vi "Settings Dialog.vi"(8 "error in (no error)":errorcluster, 11 "Settings in":T1={"Hardware Configuration"={"DAQmx Channel"="", "Max Input"=10.0, "Min Input"=-10.0, "Sample Rate"=1000.0, "DAQmx Task"=""}, "Logging Configuration"={"Log File Base Path"=path "", "TDMS File Reference"=refnum, "Samples to Save"=0, "Trigger - Time"=0, "Trigger - Threshold"=0.0, "Trigger - Channel"=0, "Enable Time Trigger"=FALSE, "Enable Threshold Trigger"=FALSE, "Always Log"=FALSE}}) -> (0 "error out":errorcluster, 1 "Cancelled?":bool=TRUE, 2 "UI Refresh Needed?":bool, 3 "Settings out":T1={"Hardware Configuration"={"DAQmx Channel"="", "Max Input"=10.0, "Min Input"=-10.0, "Sample Rate"=1000.0, "DAQmx Task"=""}, "Logging Configuration"={"Log File Base Path"=path "C:/Users/jpassiak/Documents/LabVIEW Data/Logged Data.tdms", "TDMS File Reference"=refnum, "Samples to Save"=0, "Trigger - Time"=0, "Trigger - Threshold"=0.0, "Trigger - Channel"=0, "Enable Time Trigger"=FALSE, "Enable Threshold Trigger"=FALSE, "Always Log"=FALSE}})   [LabVIEW 2015, in "Settings.lvlib"]
doc: "Dialog for selecting user specified settings."
uses:
  Settings.lvlib
  Settings.ctl
  Acquisition/Hardware Configuration.ctl
  Logging/Logging Configuration.ctl
  <vilib>/Utility/xml.llb/Write to XML File(string).vi
  Acquisition/Acquisition.lvlib
  Logging/Logging.lvlib
panel:
  in  "Log when triggered":bool
  in  "Trigger Channel":u32
  in  "Samples to Log":u32=500 min=1
  in  "Trigger Threshold (V)":dbl=2.0
  in  "Trigger Time (min)":u32=1
  in  "Enable Threshold Trigger (V):":bool
  in  "Enable Time Trigger (min):":bool
  in  "Always Log":bool
  in  "Sample Rate":dbl=1000.0
  in  "Minimum Input":dbl=-10.0
  in  "Maximum Input":dbl=10.0
  in  "DAQmx Channel":tag="Dev1/ai0"
  in  "Log File Path":path
  in  "Cancel Button":bool
  in  "OK Button":bool
  # "Acquisition"
  # "Non visible portion of dialog (needed for connector pane)."
  # "Trigger"
  # "Logging"
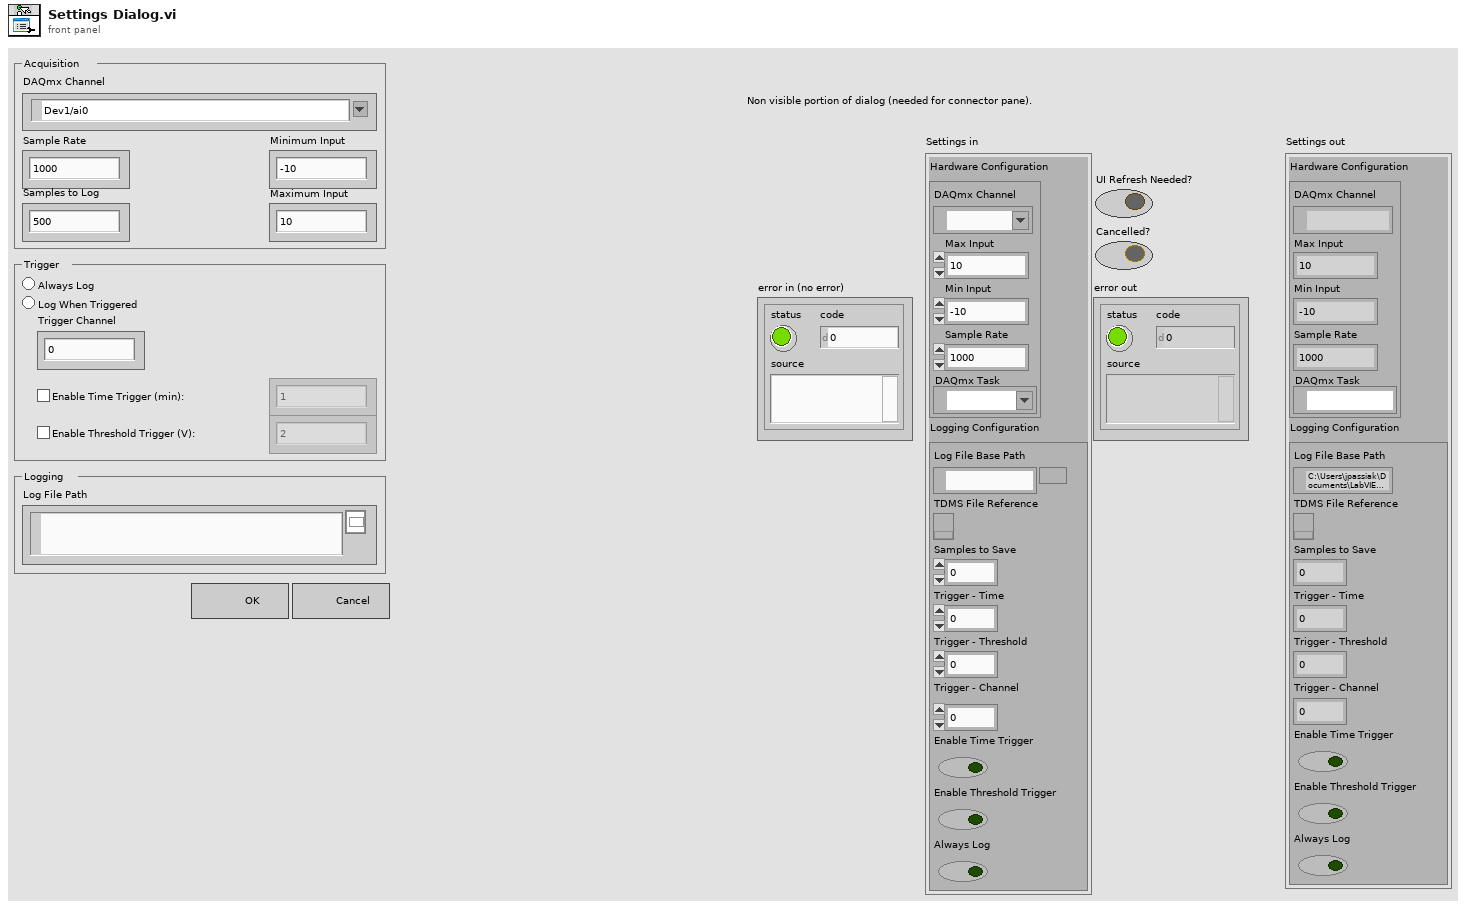
[diagram p1: front panel]
types:
  T1 = typedef "Settings.lvlib/Settings.ctl" = cluster{"Hardware Configuration":T2, "Logging Configuration":T3}
  T2 = typedef "Acquisition.lvlib/Hardware Configuration.ctl" = cluster{"DAQmx Channel":tag, "Max Input":dbl, "Min Input":dbl, "Sample Rate":dbl, "DAQmx Task":refnum<k21>}
  T3 = typedef "Logging.lvlib/Logging Configuration.ctl" = cluster{"Log File Base Path":path, "TDMS File Reference":refnum<k34>, "Samples to Save":u32, "Trigger - Time":u32, "Trigger - Threshold":dbl, "Trigger - Channel":u32, "Enable Time Trigger":bool, "Enable Threshold Trigger":bool, "Always Log":bool}
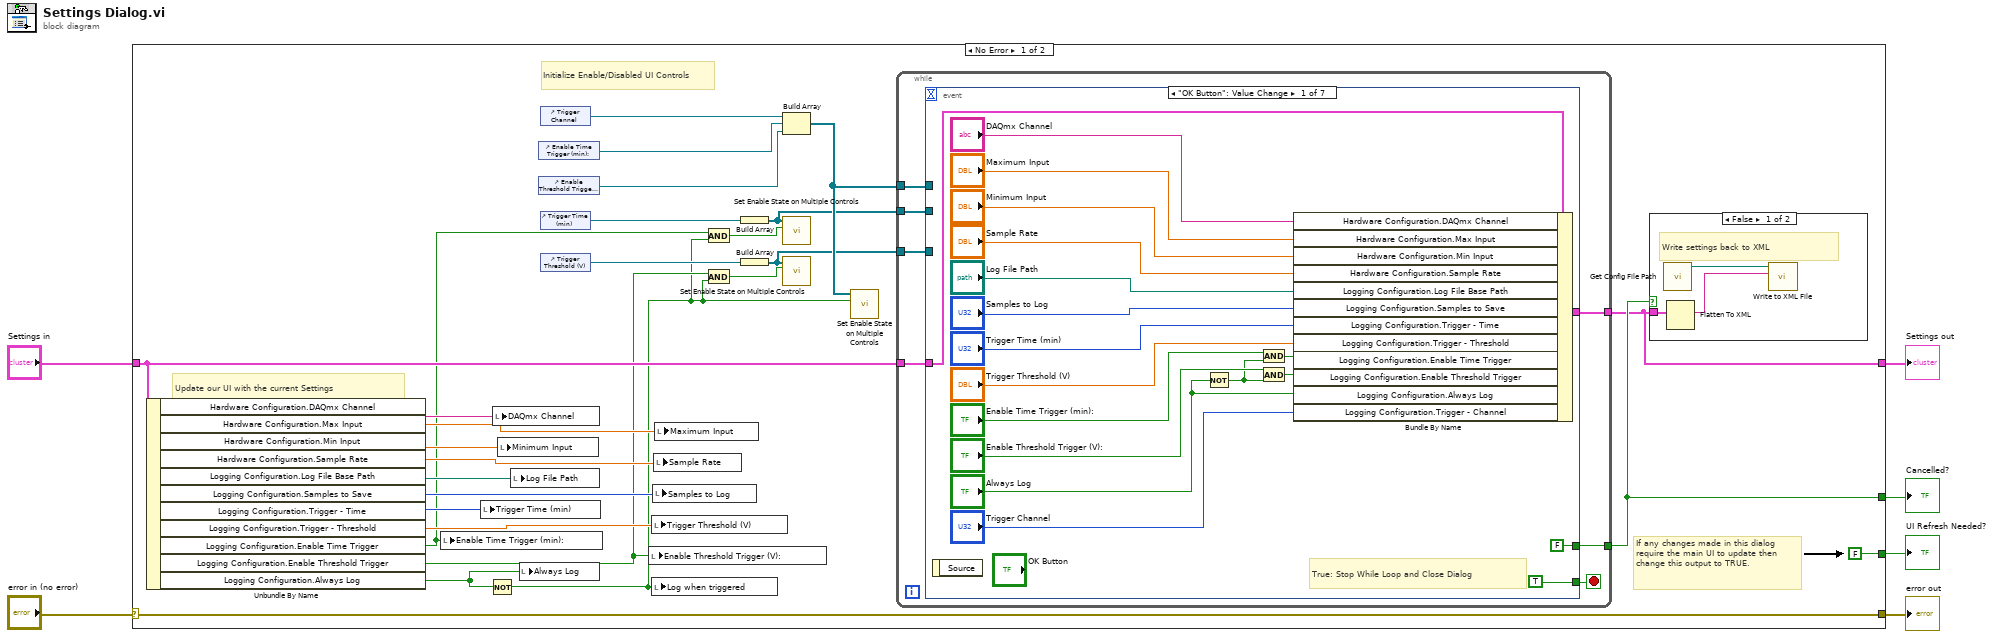
[diagram p0: block diagram]
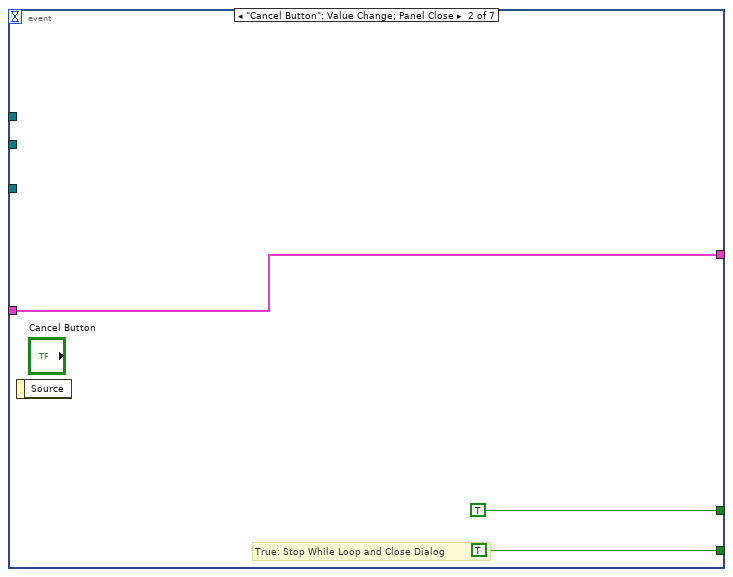
[diagram p2: hidden frame]
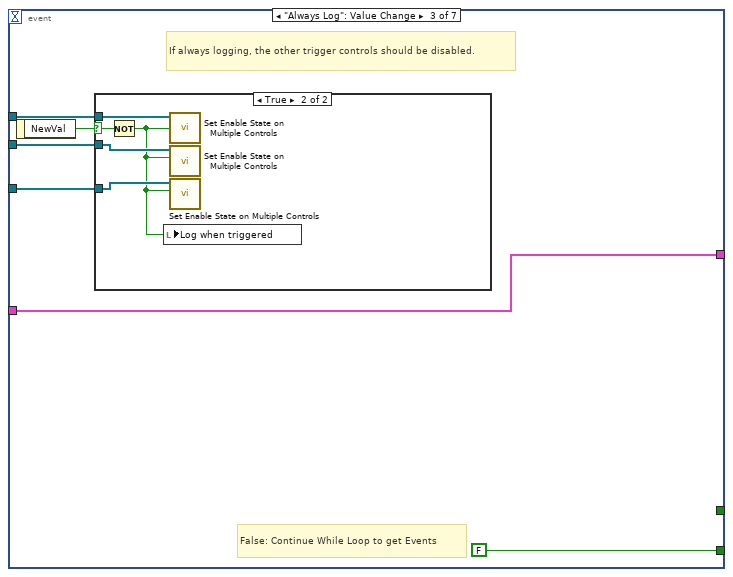
[diagram p3: hidden frame]
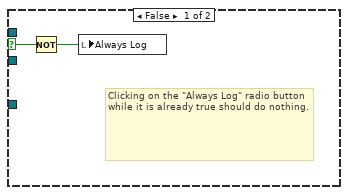
[diagram p4: hidden frame]
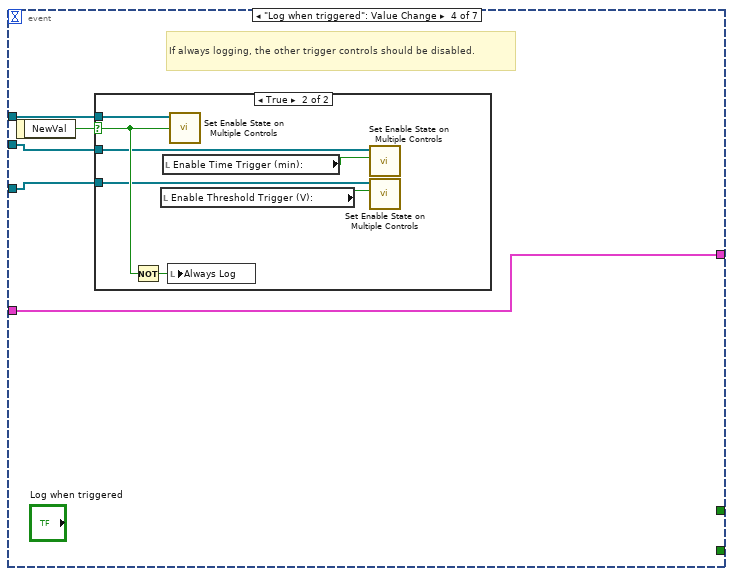
[diagram p5: hidden frame]
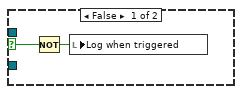
[diagram p6: hidden frame]
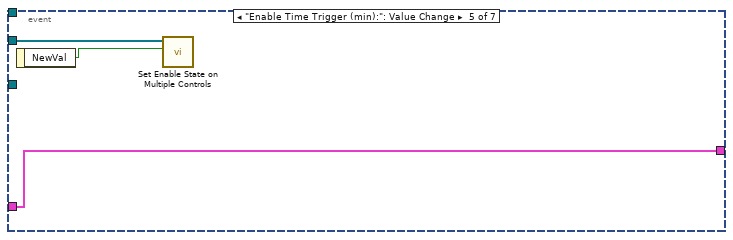
[diagram p7: hidden frame]
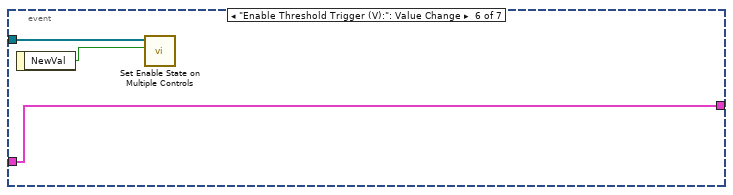
[diagram p8: hidden frame]
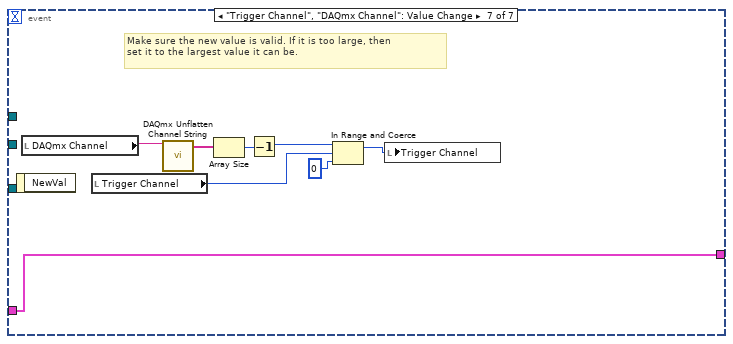
[diagram p9: hidden frame]
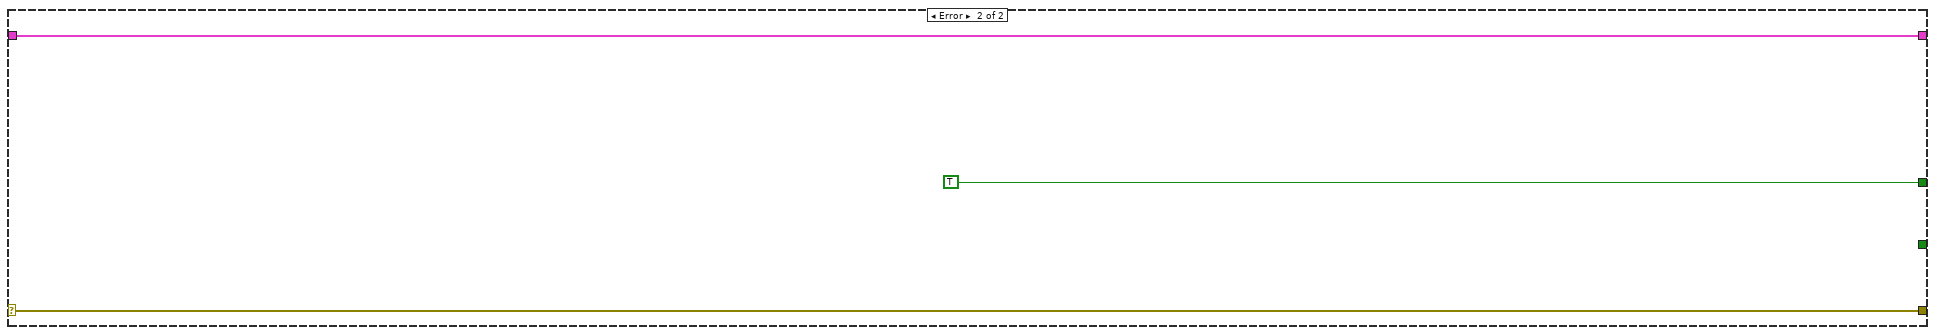
[diagram p11: hidden frame]
diagram:
  n1 = case shown="No Error" "error in (no error)" {
    selector: "error in (no error)" -> [w33 w109]
    tunnel: [w33 w109] -> w6
    tunnel: "Settings in" -> [w19 w108]
    tunnel: [w30 w108] -> w4
    tunnel: [FALSE ("UI Refresh Needed?") _] -> w3
    tunnel: [w31 TRUE ("UI Refresh Needed?")] -> w2
    frame No Error {
      # "Update our UI with the current Settings"
      # "Initialize Enable/Disabled UI Controls"
      # "If any changes made in this dialog require the main UI to update then change this output to TRUE."
      n2 = Unbundle By Name(w19) -> ("Hardware Configuration.DAQmx Channel"=w26:tag, "Hardware Configuration.Max Input"=w27:dbl, "Hardware Configuration.Min Input"=w28:dbl, "Hardware Configuration.Sample Rate"=w29:dbl, "Logging Configuration.Log File Base Path"=w25:path, "Logging Configuration.Samples to Save"=w24:u32, "Logging Configuration.Trigger - Time"=w23:u32, "Logging Configuration.Trigger - Threshold"=w22:dbl, "Logging Configuration.Enable Time Trigger"=w11:bool, "Logging Configuration.Enable Threshold Trigger"=w10:bool, "Logging Configuration.Always Log"=w21:bool)
      n3 = local write "Enable Time Trigger (min):"(w11) -> ()
      n4 = local write "Trigger Time (min)"(w23) -> ()
      n5 = Not(x=w21) -> (.not. x?=w7:bool)
      n6 = local write "DAQmx Channel"(w26) -> ()
      n7 = local write "Minimum Input"(w28) -> ()
      n8 = local write "Log File Path"(w25) -> ()
      n9 = local write "Always Log"(w21) -> ()
      n10 = control-ref of="Enable Time Trigger (min):"() -> (w17:refnum<vi>)
      n11 = control-ref of="Enable Threshold Trigger (V):"() -> (w16:refnum<vi>)
      n12 = control-ref of="Trigger Channel"() -> (w18:refnum<vi>)
      n13 = control-ref of="Trigger Time (min)"() -> (w15:refnum<vi>)
      n14 = control-ref of="Trigger Threshold (V)"() -> (w14:refnum<vi>)
      n15 = local write "Enable Threshold Trigger (V):"(w10) -> ()
      n16 = local write "Trigger Threshold (V)"(w22) -> ()
      n17 = local write "Log when triggered"(w7) -> ()
      n18 = local write "Samples to Log"(w24) -> ()
      n19 = local write "Sample Rate"(w29) -> ()
      n20 = local write "Maximum Input"(w27) -> ()
      n21 = And(x=w11, y=w7) -> (x .and. y?=w13:bool)
      n22 = And(x=w10, y=w7) -> (x .and. y?=w12:bool)
      n23 = Build Array(w15) -> (w9:refnum<vi>[])
      n24 = Build Array(w14) -> (w8:refnum<vi>[])
      n25 = Build Array(w18, w17, w16) -> (w20:refnum<vi>[])
      n26 = call "Set Enable State on Multiple Controls.vi"("Enable?"=w13, "Controls"=w9) -> ()  [unwired: 10 in]
      n27 = call "Set Enable State on Multiple Controls.vi"("Enable?"=w12, "Controls"=w8) -> ()  [unwired: 10 in]
      n28 = call "Set Enable State on Multiple Controls.vi"("Enable?"=w7, "Controls"=w20) -> ()  [unwired: 10 in]
      n29 = while {
        tunnel: [w40] -> w31
        tunnel: [w39] -> w30
        tunnel: w19 -> [w38]
        tunnel: w20 -> [w36]
        tunnel: w9 -> [w35]
        tunnel: w8 -> [w34]
        stop <- w37 stop-if-true
        n30 = event shown="[0] \"OK Button\": Value Change" {
          selector: _ -> [_ _ _ _ _ _ _]
          dyn-events: _ -> [_ _ _ _ _ _ _]
          timeout: _ -> [_ _ _ _ _ _ _]
          tunnel: [w57 w62 w68 w80 w92 w95 w103] -> w39
          tunnel: w38 -> [w56 w62 w68 w80 w92 w95 w103]
          tunnel: [FALSE ("UI Refresh Needed?") TRUE ("UI Refresh Needed?") _ _ _ _ _] -> w40
          tunnel: [TRUE TRUE FALSE _ _ _ _] -> w37
          tunnel: w36 -> [_ _ w66 w79 _ _ _]
          tunnel: w35 -> [_ _ w64 w77 w91 _ _]
          tunnel: w34 -> [_ _ w63 w76 _ w94 _]
          event "OK Button": Value Change {
            # "True: Stop While Loop and Close Dialog"
            n31 = event-data() -> ()  [unwired: 1 in, 1 out]
            n32 = Not(x="Always Log") -> (.not. x?=w41:bool)
            n33 = And(x="Enable Time Trigger (min):", y=w41) -> (x .and. y?=w42:bool)
            n34 = And(x="Enable Threshold Trigger (V):", y=w41) -> (x .and. y?=w44:bool)
            n35 = Bundle By Name(cluster=w56, "Hardware Configuration.DAQmx Channel"="DAQmx Channel", "Hardware Configuration.Max Input"="Maximum Input", "Hardware Configuration.Min Input"="Minimum Input", "Hardware Configuration.Sample Rate"="Sample Rate", "Logging Configuration.Log File Base Path"="Log File Path", "Logging Configuration.Samples to Save"="Samples to Log", "Logging Configuration.Trigger - Time"="Trigger Time (min)", "Logging Configuration.Trigger - Threshold"="Trigger Threshold (V)", "Logging Configuration.Enable Time Trigger"=w42, "Logging Configuration.Enable Threshold Trigger"=w44, "Logging Configuration.Always Log"="Always Log", "Logging Configuration.Trigger - Channel"="Trigger Channel") -> (w57:T1)
          }
          event "Cancel Button": Value Change; Panel Close {
            # "True: Stop While Loop and Close Dialog"
            n36 = event-data() -> ()  [unwired: 1 in, 1 out]
          }
          event "Always Log": Value Change {
            # "False: Continue While Loop to get Events"
            # "If always logging, the other trigger controls should be disabled."
            n37 = event-data() -> ("NewVal"=w65:bool)  [unwired: 1 in]
            n38 = case shown="True" w65 {
              selector: w65 -> [w70 w75]
              tunnel: w66 -> [_ w74]
              tunnel: w64 -> [_ w73]
              tunnel: w63 -> [_ w72]
              frame False {
                # "Clicking on the \"Always Log\" radio button while it is already true should do nothing."
                n39 = Not(x=w70) -> (.not. x?=w69:bool)
                n40 = local write "Always Log"(w69) -> ()
              }
              frame True {
                n41 = Not(x=w75) -> (.not. x?=w71:bool)
                n42 = local write "Log when triggered"(w71) -> ()
                n43 = call "Set Enable State on Multiple Controls.vi"("Enable?"=w71, "Controls"=w74) -> ()  [unwired: 10 in]
                n44 = call "Set Enable State on Multiple Controls.vi"("Enable?"=w71, "Controls"=w73) -> ()  [unwired: 10 in]
                n45 = call "Set Enable State on Multiple Controls.vi"("Enable?"=w71, "Controls"=w72) -> ()  [unwired: 10 in]
              }
            }
          }
          event "Log when triggered": Value Change {
            # "If always logging, the other trigger controls should be disabled."
            n46 = event-data() -> ("NewVal"=w78:bool)  [unwired: 1 in]
            n47 = case shown="True" w78 {
              selector: w78 -> [w82 w88]
              tunnel: w79 -> [_ w89]
              tunnel: w77 -> [_ w86]
              tunnel: w76 -> [_ w85]
              frame False {
                n48 = Not(x=w82) -> (.not. x?=w81:bool)
                n49 = local write "Log when triggered"(w81) -> ()
              }
              frame True {
                n50 = Not(x=w88) -> (.not. x?=w87:bool)
                n51 = local read "Enable Threshold Trigger (V):"() -> (w84:bool)
                n52 = local read "Enable Time Trigger (min):"() -> (w83:bool)
                n53 = local write "Always Log"(w87) -> ()
                n54 = call "Set Enable State on Multiple Controls.vi"("Enable?"=w88, "Controls"=w89) -> ()  [unwired: 10 in]
                n55 = call "Set Enable State on Multiple Controls.vi"("Enable?"=w83, "Controls"=w86) -> ()  [unwired: 10 in]
                n56 = call "Set Enable State on Multiple Controls.vi"("Enable?"=w84, "Controls"=w85) -> ()  [unwired: 10 in]
              }
            }
          }
          event "Enable Time Trigger (min):": Value Change {
            n57 = event-data() -> ("NewVal"=w90:bool)  [unwired: 1 in]
            n58 = call "Set Enable State on Multiple Controls.vi"("Enable?"=w90, "Controls"=w91) -> ()  [unwired: 10 in]
          }
          event "Enable Threshold Trigger (V):": Value Change {
            n59 = event-data() -> ("NewVal"=w93:bool)  [unwired: 1 in]
            n60 = call "Set Enable State on Multiple Controls.vi"("Enable?"=w93, "Controls"=w94) -> ()  [unwired: 10 in]
          }
          event "Trigger Channel", "DAQmx Channel": Value Change {
            # "Make sure the new value is valid. If it is too large, then\nset it to the largest value it can be."
            n61 = event-data() -> ()  [unwired: 1 in, 1 out]
            n62 = local read "DAQmx Channel"() -> (w102:tag)
            n63 = local read "Trigger Channel"() -> (w96:u32)
            n64 = call <vilib>:"DAQmx Unflatten Channel String.vi"("names in"=w102) -> ("names out"=w101:string[])  [unwired: 13 in, 1 out]
            n65 = Array Size(array=w101) -> (size(s)=w100:i32)
            n66 = Decrement(x=w100) -> (x-1=w99:i32)
            n67 = In Range and Coerce(upper limit=w99, x=w96, lower limit=u32 0) -> (coerced(x)=w97:u32)  [unwired: 1 out]
            n68 = local write "Trigger Channel"(w97) -> ()
          }
        }
      }
      n69 = case shown="False" w31 {
        tunnel: w30 -> [w105 _]
        frame False {
          # "Write settings back to XML"
          n70 = call "Get Config File Path.vi"() -> ("XML File Path"=w106:path)  [unwired: 10 in, 1 out]
          n71 = Flatten To XML(anything=w105) -> (xml string=w104:string)
          n72 = call-poly <vilib>:"Write to XML File.vi"("XML Input"=w104, "XML File Path"=w106) -> ()  [unwired: 7 in, 3 out]
        }
        frame True {
        }
      }
    }
    frame Error {
    }
  }
  "UI Refresh Needed?" <- w3
  "error out" <- w6
  "Settings out" <- w4
  "Cancelled?" <- w2
